vi "VISJS Viewer.vi"(4 "Extra Scripts":string, 5 "FileDependency out":map{path, T1}(c390), 6 "Options":string, 7 "OpenWebBrowser(False)":bool, 8 "error in":errorcluster, 9 "Embedd VISJS Librarya in HTMl File(False)":bool, 10 "HTMLFilePath":path, 11 "LibraryDependency":map{path, T3}(c390)) -> (0 "error out":errorcluster, 3 "HTMLFileContent":string)   [LabVIEW 2020, in "VISJS Viewer.lvlib"] (continued)
Hs=ig,Xs=qg,Js=sC,qs=Ug,$s=_s,ga=qs(\"string-to-symbol-registry\"),ta=qs(\"symbol-to-string-registry\");Ks({target:\"Symbol\",stat:!0,forced:!$s},{for:function(g){var t=Js(g);if(Xs(ga,t))return ga[t];var A=Hs(\"Symbol\")(t);return ga[t]=A,ta[A]=t,A}});var Aa=TA,ea=qg,Ca=xg,Ia=Og,ia=_s,oa=Ug(\"symbol-to-string-registry\");Aa({target:\"Symbol\",stat:!0,forced:!ia},{keyFor:function(g){if(!Ca(g))throw new TypeError(Ia(g)+\" is not a symbol\");if(ea(oa,g))return oa[g]}});var na=En,ra=O,sa=y,aa=sC,da=u([].push),ha=TA,la=ig,ca=a,ua=P,pa=u,fa=I,va=O,ya=xg,ma=ve,ba=function(g){if(ra(g))return g;if(na(g)){for(var t=g.length,A=[],e=0;e<t;e++){var C=g[e];\"string\"==typeof C?da(A,C):\"number\"!=typeof C&&\"Number\"!==sa(C)&&\"String\"!==sa(C)||da(A,aa(C))}var I=A.length,i=!0;return function(g,t){if(i)return i=!1,t;if(na(this))return t;for(var e=0;e<I;e++)if(A[e]===g)return t}}},wa=vg,ka=String,xa=la(\"JSON\",\"stringify\"),Ea=pa(/./.exec),Oa=pa(\"\".charAt),Ta=pa(\"\".charCodeAt),Da=pa(\"\".replace),Na=pa(1..toString),Ra=/[\\uD800-\\uDFFF]/g,Pa=/^[\\uD800-\\uDBFF]$/,Ma=/^[\\uDC00-\\uDFFF]$/,Ba=!wa||fa((function(){var g=la(\"Symbol\")(\"stringify detection\");return\"[null]\"!==xa([g])||\"{}\"!==xa({a:g})||\"{}\"!==xa(Object(g))})),za=fa((function(){return'\"\\\\udf06\\\\ud834\"'!==xa(\"\\udf06\\ud834\")||'\"\\\\udead\"'!==xa(\"\\udead\")})),Sa=function(g,t){var A=ma(arguments),e=ba(t);if(va(e)||void 0!==g&&!ya(g))return A[1]=function(g,t){if(va(e)&&(t=ua(e,this,ka(g),t)),!ya(t))return t},ca(xa,null,A)},Za=function(g,t,A){var e=Oa(A,t-1),C=Oa(A,t+1);return Ea(Pa,g)&&!Ea(Ma,C)||Ea(Ma,g)&&!Ea(Pa,e)?\"\\\\u\"+Na(Ta(g,0),16):g};xa&&ha({target:\"JSON\",stat:!0,arity:3,forced:Ba||za},{stringify:function(g,t,A){var e=ma(arguments),C=ca(Ba?Sa:xa,null,e);return za&&\"string\"==typeof C?Da(C,Ra,Za):C}});var Fa=ee,Ga=Hg;TA({target:\"Object\",stat:!0,forced:!vg||I((function(){Fa.f(1)}))},{getOwnPropertySymbols:function(g){var t=Fa.f;return t?t(Ga(g)):[]}}),wr(\"asyncIterator\"),wr(\"hasInstance\"),wr(\"isConcatSpreadable\"),wr(\"iterator\"),wr(\"match\"),wr(\"matchAll\"),wr(\"replace\"),wr(\"search\"),wr(\"species\"),wr(\"split\");var ja=Tr;wr(\"toPrimitive\"),ja();var La=ig,Va=_I;wr(\"toStringTag\"),Va(La(\"Symbol\"),\"Symbol\"),wr(\"unscopables\"),_I(C.JSON,\"JSON\",!0);var Ya=tg.Symbol,Wa=dt,Qa=Jt.f,Ua=Wa(\"metadata\"),_a=Function.prototype;void 0===_a[Ua]&&Qa(_a,Ua,{value:null}),wr(\"asyncDispose\"),wr(\"dispose\"),wr(\"metadata\");var Ka=Ya,Ha=u,Xa=ig(\"Symbol\"),Ja=Xa.keyFor,qa=Ha(Xa.prototype.valueOf),$a=Xa.isRegisteredSymbol||function(g){try{return void 0!==Ja(qa(g))}catch(g){return!1}};TA({target:\"Symbol\",stat:!0},{isRegisteredSymbol:$a});for(var gd=Ug,td=ig,Ad=u,ed=xg,Cd=dt,Id=td(\"Symbol\"),id=Id.isWellKnownSymbol,od=td(\"Object\",\"getOwnPropertyNames\"),nd=Ad(Id.prototype.valueOf),rd=gd(\"wks\"),sd=0,ad=od(Id),dd=ad.length;sd<dd;sd++)try{var hd=ad[sd];ed(Id[hd])&&Cd(hd)}catch(g){}var ld=function(g){if(id&&id(g))return!0;try{for(var t=nd(g),A=0,e=od(rd),C=e.length;A<C;A++)if(rd[e[A]]==t)return!0}catch(g){}return!1};TA({target:\"Symbol\",stat:!0,forced:!0},{isWellKnownSymbol:ld}),wr(\"matcher\"),wr(\"observable\"),TA({target:\"Symbol\",stat:!0,name:\"isRegisteredSymbol\"},{isRegistered:$a}),TA({target:\"Symbol\",stat:!0,name:\"isWellKnownSymbol\",forced:!0},{isWellKnown:ld}),wr(\"metadataKey\"),wr(\"patternMatch\"),wr(\"replaceAll\");var cd=Ka,ud=A(cd),pd=pr.f(\"iterator\"),fd=pd,vd=A(fd);function yd(g){return yd=\"function\"==typeof ud&&\"symbol\"==typeof vd?function(g){return typeof g}:function(g){return g&&\"function\"==typeof ud&&g.constructor===ud&&g!==ud.prototype?\"symbol\":typeof g},yd(g)}var md=A(pr.f(\"toPrimitive\"));function bd(g){var t=function(g,t){if(\"object\"!==yd(g)||null===g)return g;var A=g[md];if(void 0!==A){var e=A.call(g,t||\"default\");if(\"object\"!==yd(e))return e;throw new TypeError(\"@@toPrimitive must return a primitive value.\")}return(\"string\"===t?String:Number)(g)}(g,\"string\");return\"symbol\"===yd(t)?t:String(t)}function wd(g,t){for(var A=0;A<t.length;A++){var e=t[A];e.enumerable=e.enumerable||!1,e.configurable=!0,\"value\"in e&&(e.writable=!0),kn(g,bd(e.key),e)}}function kd(g,t,A){return t&&wd(g.prototype,t),A&&wd(g,A),kn(g,\"prototype\",{writable:!1}),g}TA({target:\"Array\",stat:!0},{isArray:En});var xd=tg.Array.isArray,Ed=A(xd);var Od=D,Td=En,Dd=TypeError,Nd=Object.getOwnPropertyDescriptor,Rd=Od&&!function(){if(void 0!==this)return!0;try{Object.defineProperty([],\"length\",{writable:!1}).length=1}catch(g){return g instanceof TypeError}}()?function(g,t){if(Td(g)&&!Nd(g,\"length\").writable)throw new Dd(\"Cannot set read only .length\");return g.length=t}:function(g,t){return g.length=t},Pd=Hg,Md=jA,Bd=Rd,zd=Tn;TA({target:\"Array\",proto:!0,arity:1,forced:I((function(){return 4294967297!==[].push.call({length:4294967296},1)}))||!function(){try{Object.defineProperty([],\"length\",{writable:!1}).push()}catch(g){return g instanceof TypeError}}()},{push:function(g){var t=Pd(this),A=Md(t),e=arguments.length;zd(A+e);for(var C=0;C<e;C++)t[A]=arguments[C],A++;return Bd(t,A),A}});var Sd=Me(\"Array\").push,Zd=og,Fd=Sd,Gd=Array.prototype,jd=function(g){var t=g.push;return g===Gd||Zd(Gd,g)&&t===Gd.push?Fd:t},Ld=jd,Vd=A(Ld);var Yd=TA,Wd=En,Qd=ro,Ud=gg,_d=SA,Kd=jA,Hd=J,Xd=lo,Jd=dt,qd=ve,$d=Gn(\"slice\"),gh=Jd(\"species\"),th=Array,Ah=Math.max;Yd({target:\"Array\",proto:!0,forced:!$d},{slice:function(g,t){var A,e,C,I=Hd(this),i=Kd(I),o=_d(g,i),n=_d(void 0===t?i:t,i);if(Wd(I)&&(A=I.constructor,(Qd(A)&&(A===th||Wd(A.prototype))||Ud(A)&&null===(A=A[gh]))&&(A=void 0),A===th||void 0===A))return qd(I,o,n);for(e=new(void 0===A?th:A)(Ah(n-o,0)),C=0;o<n;o++,C++)o in I&&Xd(e,C,I[o]);return e.length=C,e}});var eh=Me(\"Array\").slice,Ch=og,Ih=eh,ih=Array.prototype,oh=function(g){var t=g.slice;return g===ih||Ch(ih,g)&&t===ih.slice?Ih:t},nh=oh,rh=nh,sh=A(rh),ah=A(Qo);function dh(g,t){(null==t||t>g.length)&&(t=g.length);for(var A=0,e=new Array(t);A<t;A++)e[A]=g[A];return e}function hh(g,t){var A;if(g){if(\"string\"==typeof g)return dh(g,t);var e=sh(A=Object.prototype.toString.call(g)).call(A,8,-1);return\"Object\"===e&&g.constructor&&(e=g.constructor.name),\"Map\"===e||\"Set\"===e?ah(g):\"Arguments\"===e||/^(?:Ui|I)nt(?:8|16|32)(?:Clamped)?Array$/.test(e)?dh(g,t):void 0}}function lh(g,t){return function(g){if(Ed(g))return g}(g)||function(g,t){var A=null==g?null:void 0!==ud&&hn(g)||g[\"@@iterator\"];if(null!=A){var e,C,I,i,o=[],n=!0,r=!1;try{if(I=(A=A.call(g)).next,0===t){if(Object(A)!==A)return;n=!1}else for(;!(n=(e=I.call(A)).done)&&(Vd(o).call(o,e.value),o.length!==t);n=!0);}catch(g){r=!0,C=g}finally{try{if(!n&&null!=A.return&&(i=A.return(),Object(i)!==i))return}finally{if(r)throw C}}return o}}(g,t)||hh(g,t)||function(){throw new TypeError(\"Invalid attempt to destructure non-iterable instance.\\nIn order to be iterable, non-array objects must have a [Symbol.iterator]() method.\")}()}function ch(g){return function(g){if(Ed(g))return dh(g)}(g)||function(g){if(void 0!==ud&&null!=hn(g)||null!=g[\"@@iterator\"])return ah(g)}(g)||hh(g)||function(){throw new TypeError(\"Invalid attempt to spread non-iterable instance.\\nIn order to be iterable, non-array objects must have a [Symbol.iterator]() method.\")}()}var uh=A(Ya),ph=Me(\"Array\").concat,fh=og,vh=ph,yh=Array.prototype,mh=function(g){var t=g.concat;return g===yh||fh(yh,g)&&t===yh.concat?vh:t},bh=A(mh),wh=A(nh),kh=ig,xh=gr,Eh=ee,Oh=AA,Th=u([].concat),Dh=kh(\"Reflect\",\"ownKeys\")||function(g){var t=xh.f(Oh(g)),A=Eh.f;return A?Th(t,A(g)):t};TA({target:\"Reflect\",stat:!0},{ownKeys:Dh});var Nh=A(tg.Reflect.ownKeys),Rh=A(xd),Ph=Sr.map;TA({target:\"Array\",proto:!0,forced:!Gn(\"map\")},{map:function(g){return Ph(this,g,arguments.length>1?arguments[1]:void 0)}});var Mh=Me(\"Array\").map,Bh=og,zh=Mh,Sh=Array.prototype,Zh=function(g){var t=g.map;return g===Sh||Bh(Sh,g)&&t===Sh.map?zh:t},Fh=A(Zh),Gh=Hg,jh=Ae;TA({target:\"Object\",stat:!0,forced:I((function(){jh(1)}))},{keys:function(g){return jh(Gh(g))}});var Lh=A(tg.Object.keys),Vh=TA,Yh=Date,Wh=u(Yh.prototype.getTime);Vh({target:\"Date\",stat:!0},{now:function(){return Wh(new Yh)}});var Qh=A(tg.Date.now),Uh=I,_h=function(g,t){var A=[][g];return!!A&&Uh((function(){A.call(null,t||function(){return 1},1)}))},Kh=Sr.forEach,Hh=_h(\"forEach\")?[].forEach:function(g){return Kh(this,g,arguments.length>1?arguments[1]:void 0)};TA({target:\"Array\",proto:!0,forced:[].forEach!==Hh},{forEach:Hh});var Xh=Me(\"Array\").forEach,Jh=oC,qh=qg,$h=og,gl=Xh,tl=Array.prototype,Al={DOMTokenList:!0,NodeList:!0},el=function(g){var t=g.forEach;return g===tl||$h(tl,g)&&t===tl.forEach||qh(Al,Jh(g))?gl:t},Cl=A(el),Il=TA,il=En,ol=u([].reverse),nl=[1,2];Il({target:\"Array\",proto:!0,forced:String(nl)===String(nl.reverse())},{reverse:function(){return il(this)&&(this.length=this.length),ol(this)}});var rl=Me(\"Array\").reverse,sl=og,al=rl,dl=Array.prototype,hl=function(g){var t=g.reverse;return g===dl||sl(dl,g)&&t===dl.reverse?al:t},ll=hl,cl=A(ll),ul=Og,pl=TypeError,fl=function(g,t){if(!delete g[t])throw new pl(\"Cannot delete property \"+ul(t)+\" of \"+ul(g))},vl=TA,yl=Hg,ml=SA,bl=PA,wl=jA,kl=Rd,xl=Tn,El=zn,Ol=lo,Tl=fl,Dl=Gn(\"splice\"),Nl=Math.max,Rl=Math.min;vl({target:\"Array\",proto:!0,forced:!Dl},{splice:function(g,t){var A,e,C,I,i,o,n=yl(this),r=wl(n),s=ml(g,r),a=arguments.length;for(0===a?A=e=0:1===a?(A=0,e=r-s):(A=a-2,e=Rl(Nl(bl(t),0),r-s)),xl(r+A-e),C=El(n,e),I=0;I<e;I++)(i=s+I)in n&&Ol(C,I,n[i]);if(C.length=e,A<e){for(I=s;I<r-e;I++)o=I+A,(i=I+e)in n?n[o]=n[i]:Tl(n,o);for(I=r;I>r-e+A;I--)Tl(n,I-1)}else if(A>e)for(I=r-e;I>s;I--)o=I+A-1,(i=I+e-1)in n?n[o]=n[i]:Tl(n,o);for(I=0;I<A;I++)n[I+s]=arguments[I+2];return kl(n,r-e+A),C}});var Pl=Me(\"Array\").splice,Ml=og,Bl=Pl,zl=Array.prototype,Sl=function(g){var t=g.splice;return g===zl||Ml(zl,g)&&t===zl.splice?Bl:t},Zl=A(Sl),Fl=QA.includes;TA({target:\"Array\",proto:!0,forced:I((function(){return!Array(1).includes()}))},{includes:function(g){return Fl(this,g,arguments.length>1?arguments[1]:void 0)}});var Gl=Me(\"Array\").includes,jl=gg,Ll=y,Vl=dt(\"match\"),Yl=function(g){var t;return jl(g)&&(void 0!==(t=g[Vl])?!!t:\"RegExp\"===Ll(g))},Wl=TypeError,Ql=dt(\"match\"),Ul=TA,_l=function(g){if(Yl(g))throw new Wl(\"The method doesn't accept regular expressions\");return g},Kl=K,Hl=sC,Xl=function(g){var t=/./;try{\"/./\"[g](t)}catch(A){try{return t[Ql]=!1,\"/./\"[g](t)}catch(g){}}return!1},Jl=u(\"\".indexOf);Ul({target:\"String\",proto:!0,forced:!Xl(\"includes\")},{includes:function(g){return!!~Jl(Hl(Kl(this)),Hl(_l(g)),arguments.length>1?arguments[1]:void 0)}});var ql=Me(\"String\").includes,$l=og,gc=Gl,tc=ql,Ac=Array.prototype,ec=String.prototype,Cc=function(g){var t=g.includes;return g===Ac||$l(Ac,g)&&t===Ac.includes?gc:\"string\"==typeof g||g===ec||$l(ec,g)&&t===ec.includes?tc:t},Ic=A(Cc),ic=Hg,oc=EI,nc=fI;TA({target:\"Object\",stat:!0,forced:I((function(){oc(1)})),sham:!nc},{getPrototypeOf:function(g){return oc(ic(g))}});var rc=tg.Object.getPrototypeOf,sc=A(rc),ac=Sr.filter;TA({target:\"Array\",proto:!0,forced:!Gn(\"filter\")},{filter:function(g){return ac(this,g,arguments.length>1?arguments[1]:void 0)}});var dc=Me(\"Array\").filter,hc=og,lc=dc,cc=Array.prototype,uc=function(g){var t=g.filter;return g===cc||hc(cc,g)&&t===cc.filter?lc:t},pc=A(uc),fc=\"\\t\\n\\v\\f\\r  ?            ? \\u2028\\u2029\\ufeff\",vc=K,yc=sC,mc=fc,bc=u(\"\".replace),wc=RegExp(\"^[\"+mc+\"]+\"),kc=RegExp(\"(^|[^\"+mc+\"])[\"+mc+\"]+$\"),xc=function(g){return function(t){var A=yc(vc(t));return 1&g&&(A=bc(A,wc,\"\")),2&g&&(A=bc(A,kc,\"$1\")),A}},Ec={start:xc(1),end:xc(2),trim:xc(3)},Oc=C,Tc=I,Dc=u,Nc=sC,Rc=Ec.trim,Pc=fc,Mc=Oc.parseInt,Bc=Oc.Symbol,zc=Bc&&Bc.iterator,Sc=/^[+-]?0x/i,Zc=Dc(Sc.exec),Fc=8!==Mc(Pc+\"08\")||22!==Mc(Pc+\"0x16\")||zc&&!Tc((function(){Mc(Object(zc))}))?function(g,t){var A=Rc(Nc(g));return Mc(A,t>>>0||(Zc(Sc,A)?16:10))}:Mc;TA({global:!0,forced:parseInt!==Fc},{parseInt:Fc});var Gc=A(tg.parseInt),jc=TA,Lc=QA.indexOf,Vc=_h,Yc=w([].indexOf),Wc=!!Yc&&1/Yc([1],1,-0)<0;jc({target:\"Array\",proto:!0,forced:Wc||!Vc(\"indexOf\")},{indexOf:function(g){var t=arguments.length>1?arguments[1]:void 0;return Wc?Yc(this,g,t)||0:Lc(this,g,t)}});var Qc=Me(\"Array\").indexOf,Uc=og,_c=Qc,Kc=Array.prototype,Hc=function(g){var t=g.indexOf;return g===Kc||Uc(Kc,g)&&t===Kc.indexOf?_c:t},Xc=A(Hc);TA({target:\"Object\",stat:!0,sham:!D},{create:pI});var Jc=tg.Object,qc=function(g,t){return Jc.create(g,t)},$c=A(qc),gu=tg,tu=a;gu.JSON||(gu.JSON={stringify:JSON.stringify});var Au=function(g,t,A){return tu(gu.JSON.stringify,null,arguments)},eu=A(Au),Cu=\"function\"==typeof Bun&&Bun&&\"string\"==typeof Bun.version,Iu=TypeError,iu=function(g,t){if(g<t)throw new Iu(\"Not enough arguments\");return g},ou=C,nu=a,ru=O,su=Cu,au=ng,du=ve,hu=iu,lu=ou.Function,cu=/MSIE .\\./.test(au)||su&&function(){var g=ou.Bun.version.split(\".\");return g.length<3||\"0\"===g[0]&&(g[1]<3||\"3\"===g[1]&&\"0\"===g[2])}(),uu=function(g,t){var A=t?2:1;return cu?function(e,C){var I=hu(arguments.length,1)>A,i=ru(e)?e:lu(e),o=I?du(arguments,A):[],n=I?function(){nu(i,this,o)}:i;return t?g(n,C):g(n)}:g},pu=TA,fu=C,vu=uu(fu.setInterval,!0);pu({global:!0,bind:!0,forced:fu.setInterval!==vu},{setInterval:vu});var yu=TA,mu=C,bu=uu(mu.setTimeout,!0);yu({global:!0,bind:!0,forced:mu.setTimeout!==bu},{setTimeout:bu});var wu=A(tg.setTimeout),ku=Hg,xu=SA,Eu=jA,Ou=function(g){for(var t=ku(this),A=Eu(t),e=arguments.length,C=xu(e>1?arguments[1]:void 0,A),I=e>2?arguments[2]:void 0,i=void 0===I?A:xu(I,A);i>C;)t[C++]=g;return t};TA({target:\"Array\",proto:!0},{fill:Ou});var Tu,Du=Me(\"Array\").fill,Nu=og,Ru=Du,Pu=Array.prototype,Mu=function(g){var t=g.fill;return g===Pu||Nu(Pu,g)&&t===Pu.fill?Ru:t},Bu=A(Mu);\n/*! Hammer.JS - v2.0.17-rc - 2019-12-16\n\t * http://naver.github.io/egjs\n\t *\n\t * Forked By Naver egjs\n\t * Copyright (c) hammerjs\n\t * Licensed under the MIT license */\nfunction zu(){return zu=Object.assign||function(g){for(var t=1;t<arguments.length;t++){var A=arguments[t];for(var e in A)Object.prototype.hasOwnProperty.call(A,e)&&(g[e]=A[e])}return g},zu.apply(this,arguments)}function Su(g,t){g.prototype=Object.create(t.prototype),g.prototype.constructor=g,g.__proto__=t}function Zu(g){if(void 0===g)throw new ReferenceError(\"this hasn't been initialised - super() hasn't been called\");return g}Tu=\"function\"!=typeof Object.assign?function(g){if(null==g)throw new TypeError(\"Cannot convert undefined or null to object\");for(var t=Object(g),A=1;A<arguments.length;A++){var e=arguments[A];if(null!=e)for(var C in e)e.hasOwnProperty(C)&&(t[C]=e[C])}return t}:Object.assign;var Fu,Gu=Tu,ju=[\"\",\"webkit\",\"Moz\",\"MS\",\"ms\",\"o\"],Lu=\"undefined\"==typeof document?{style:{}}:document.createElement(\"div\"),Vu=Math.round,Yu=Math.abs,Wu=Date.now;function Qu(g,t){for(var A,e,C=t[0].toUpperCase()+t.slice(1),I=0;I<ju.length;){if((e=(A=ju[I])?A+C:t)in g)return e;I++}}Fu=\"undefined\"==typeof window?{}:window;var Uu=Qu(Lu.style,\"touchAction\"),_u=void 0!==Uu;var Ku=\"compute\",Hu=\"auto\",Xu=\"manipulation\",Ju=\"none\",qu=\"pan-x\",$u=\"pan-y\",gp=function(){if(!_u)return!1;var g={},t=Fu.CSS&&Fu.CSS.supports;return[\"auto\",\"manipulation\",\"pan-y\",\"pan-x\",\"pan-x pan-y\",\"none\"].forEach((function(A){return g[A]=!t||Fu.CSS.supports(\"touch-action\",A)})),g}(),tp=\"ontouchstart\"in Fu,Ap=void 0!==Qu(Fu,\"PointerEvent\"),ep=tp&&/mobile|tablet|ip(ad|hone|od)|android/i.test(navigator.userAgent),Cp=\"touch\",Ip=\"mouse\",ip=25,op=1,np=4,rp=8,sp=1,ap=2,dp=4,hp=8,lp=16,cp=ap|dp,up=hp|lp,pp=cp|up,fp=[\"x\",\"y\"],vp=[\"clientX\",\"clientY\"];function yp(g,t,A){var e;if(g)if(g.forEach)g.forEach(t,A);else if(void 0!==g.length)for(e=0;e<g.length;)t.call(A,g[e],e,g),e++;else for(e in g)g.hasOwnProperty(e)&&t.call(A,g[e],e,g)}function mp(g,t){return\"function\"==typeof g?g.apply(t&&t[0]||void 0,t):g}function bp(g,t){return g.indexOf(t)>-1}var wp=function(){function g(g,t){this.manager=g,this.set(t)}var t=g.prototype;return t.set=function(g){g===Ku&&(g=this.compute()),_u&&this.manager.element.style&&gp[g]&&(this.manager.element.style[Uu]=g),this.actions=g.toLowerCase().trim()},t.update=function(){this.set(this.manager.options.touchAction)},t.compute=function(){var g=[];return yp(this.manager.recognizers,(function(t){mp(t.options.enable,[t])&&(g=g.concat(t.getTouchAction()))})),function(g){if(bp(g,Ju))return Ju;var t=bp(g,qu),A=bp(g,$u);return t&&A?Ju:t||A?t?qu:$u:bp(g,Xu)?Xu:Hu}(g.join(\" \"))},t.preventDefaults=function(g){var t=g.srcEvent,A=g.offsetDirection;if(this.manager.session.prevented)t.preventDefault();else{var e=this.actions,C=bp(e,Ju)&&!gp[Ju],I=bp(e,$u)&&!gp[$u],i=bp(e,qu)&&!gp[qu];if(C){var o=1===g.pointers.length,n=g.distance<2,r=g.deltaTime<250;if(o&&n&&r)return}if(!i||!I)return C||I&&A&cp||i&&A&up?this.preventSrc(t):void 0}},t.preventSrc=function(g){this.manager.session.prevented=!0,g.preventDefault()},g}();function kp(g,t){for(;g;){if(g===t)return!0;g=g.parentNode}return!1}function xp(g){var t=g.length;if(1===t)return{x:Vu(g[0].clientX),y:Vu(g[0].clientY)};for(var A=0,e=0,C=0;C<t;)A+=g[C].clientX,e+=g[C].clientY,C++;return{x:Vu(A/t),y:Vu(e/t)}}function Ep(g){for(var t=[],A=0;A<g.pointers.length;)t[A]={clientX:Vu(g.pointers[A].clientX),clientY:Vu(g.pointers[A].clientY)},A++;return{timeStamp:Wu(),pointers:t,center:xp(t),deltaX:g.deltaX,deltaY:g.deltaY}}function Op(g,t,A){A||(A=fp);var e=t[A[0]]-g[A[0]],C=t[A[1]]-g[A[1]];return Math.sqrt(e*e+C*C)}function Tp(g,t,A){A||(A=fp);var e=t[A[0]]-g[A[0]],C=t[A[1]]-g[A[1]];return 180*Math.atan2(C,e)/Math.PI}function Dp(g,t){return g===t?sp:Yu(g)>=Yu(t)?g<0?ap:dp:t<0?hp:lp}function Np(g,t,A){return{x:t/g||0,y:A/g||0}}function Rp(g,t){var A=g.session,e=t.pointers,C=e.length;A.firstInput||(A.firstInput=Ep(t)),C>1&&!A.firstMultiple?A.firstMultiple=Ep(t):1===C&&(A.firstMultiple=!1);var I=A.firstInput,i=A.firstMultiple,o=i?i.center:I.center,n=t.center=xp(e);t.timeStamp=Wu(),t.deltaTime=t.timeStamp-I.timeStamp,t.angle=Tp(o,n),t.distance=Op(o,n),function(g,t){var A=t.center,e=g.offsetDelta||{},C=g.prevDelta||{},I=g.prevInput||{};t.eventType!==op&&I.eventType!==np||(C=g.prevDelta={x:I.deltaX||0,y:I.deltaY||0},e=g.offsetDelta={x:A.x,y:A.y}),t.deltaX=C.x+(A.x-e.x),t.deltaY=C.y+(A.y-e.y)}(A,t),t.offsetDirection=Dp(t.deltaX,t.deltaY);var r,s,a=Np(t.deltaTime,t.deltaX,t.deltaY);t.overallVelocityX=a.x,t.overallVelocityY=a.y,t.overallVelocity=Yu(a.x)>Yu(a.y)?a.x:a.y,t.scale=i?(r=i.pointers,Op((s=e)[0],s[1],vp)/Op(r[0],r[1],vp)):1,t.rotation=i?function(g,t){return Tp(t[1],t[0],vp)+Tp(g[1],g[0],vp)}(i.pointers,e):0,t.maxPointers=A.prevInput?t.pointers.length>A.prevInput.maxPointers?t.pointers.length:A.prevInput.maxPointers:t.pointers.length,function(g,t){var A,e,C,I,i=g.lastInterval||t,o=t.timeStamp-i.timeStamp;if(t.eventType!==rp&&(o>ip||void 0===i.velocity)){var n=t.deltaX-i.deltaX,r=t.deltaY-i.deltaY,s=Np(o,n,r);e=s.x,C=s.y,A=Yu(s.x)>Yu(s.y)?s.x:s.y,I=Dp(n,r),g.lastInterval=t}else A=i.velocity,e=i.velocityX,C=i.velocityY,I=i.direction;t.velocity=A,t.velocityX=e,t.velocityY=C,t.direction=I}(A,t);var d,h=g.element,l=t.srcEvent;kp(d=l.composedPath?l.composedPath()[0]:l.path?l.path[0]:l.target,h)&&(h=d),t.target=h}function Pp(g,t,A){var e=A.pointers.length,C=A.changedPointers.length,I=t&op&&e-C==0,i=t&(np|rp)&&e-C==0;A.isFirst=!!I,A.isFinal=!!i,I&&(g.session={}),A.eventType=t,Rp(g,A),g.emit(\"hammer.input\",A),g.recognize(A),g.session.prevInput=A}function Mp(g){return g.trim().split(/\\s+/g)}function Bp(g,t,A){yp(Mp(t),(function(t){g.addEventListener(t,A,!1)}))}function zp(g,t,A){yp(Mp(t),(function(t){g.removeEventListener(t,A,!1)}))}function Sp(g){var t=g.ownerDocument||g;return t.defaultView||t.parentWindow||window}var Zp=function(){function g(g,t){var A=this;this.manager=g,this.callback=t,this.element=g.element,this.target=g.options.inputTarget,this.domHandler=function(t){mp(g.options.enable,[g])&&A.handler(t)},this.init()}var t=g.prototype;return t.handler=function(){},t.init=function(){this.evEl&&Bp(this.element,this.evEl,this.domHandler),this.evTarget&&Bp(this.target,
